vi "PlotObject_Excists.vi"(1 "PlotName":string) -> (0 "found?":bool)   [LabVIEW 2017]
doc: "Checks whether the PlotObject with the name \"PlotName\" excists.\nCan be used to check whether PlotWindow is open already and doesn't need\nto be opened again.\n\nIn MSControl PlotName = IsotopeName.\nIn MSEval PlotName = SessionID_IsotopeName"
uses:
  global_variables.vi
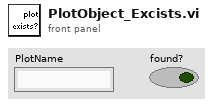
[diagram p1: front panel]
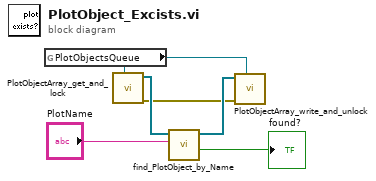
[diagram p0: block diagram]
diagram:
  n1 = global read "global_variables.vi" "PlotObjectsQueue"() -> (w2:refnum<queue>)
  n2 = call "PlotObjectArray_get_and_lock.vi"("External PlotObjQueue in"=w2) -> ("error out"=w3:errorcluster, "PlotObjects"=w5:refnum<class "Plots.lvclass">[])  [unwired: 9 in]
  n3 = call "find_PlotObject_by_Name.vi"("Plot Name/ID"="PlotName", "PlotObj Array in"=w5) -> ("found?"=→"found?":bool, "PlotObj Array out"=w4:refnum<class "Plots.lvclass">[])  [unwired: 6 in, 2 out]
  n4 = call "PlotObjectArray_write_and_unlock.vi"("External PlotObjQueue in"=w2, "error in (no error)"=w3, "PlotObjects"=w4) -> ()  [unwired: 8 in, 1 out]
